vi "SetXMenuData.vi"(8 "error in (no error)":errorcluster, 9 "Items":T1(array[cluster]), 11 "CMenu in":refnum<class "CMenu.lvclass">) -> (0 "error out":errorcluster, 3 "CMenu out":refnum<class "CMenu.lvclass">)   [LabVIEW 2020, in "CMenu.lvclass"]
uses:
  CMenu.lvclass
  CMenu.lvclass/CMenu.ctl
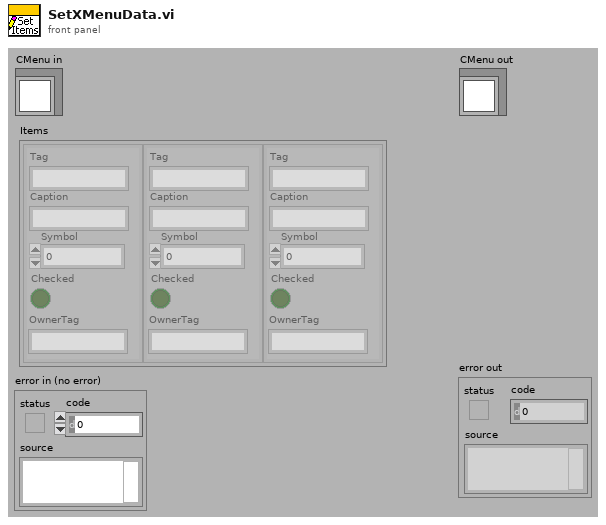
[diagram p1: front panel]
types:
  T1 = cluster{"Tag":string, "Caption":string, "Symbol":i32, "Checked":bool, "OwnerTag":string}[]
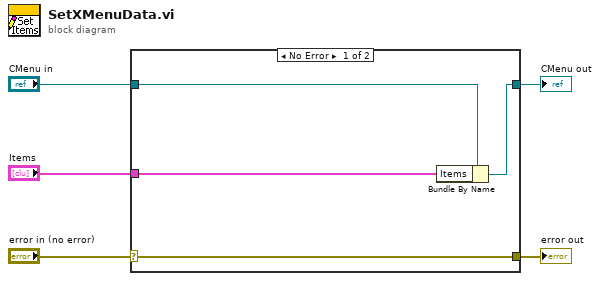
[diagram p0: block diagram]
diagram:
  n1 = case shown="No Error" "error in (no error)" {
    selector: "error in (no error)" -> [w9 w10]
    tunnel: [w9 w10] -> w4
    tunnel: [w7 w11] -> w2
    tunnel: "CMenu in" -> [w8 w11]
    tunnel: "Items" -> [w6 _]
    frame No Error {
      n2 = Bundle By Name(cluster=w8, "Items"=w6) -> (w7:refnum<class "CMenu.lvclass">)
    }
    frame Error {
    }
  }
  "error out" <- w4
  "CMenu out" <- w2
